vi "num2stringArr.vi"(0 "item 1":dbl, 1 "item 2":dbl, 2 "item 3":dbl, 3 "item 4":dbl, 4 "item5":dbl) -> (5 "Array":string[][](array[string]))   [LabVIEW 2015]
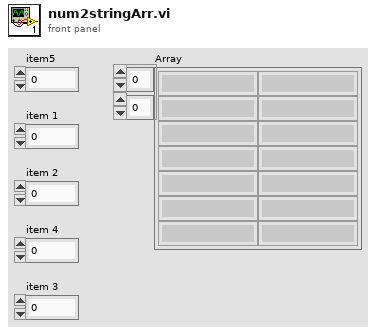
[diagram p1: front panel]
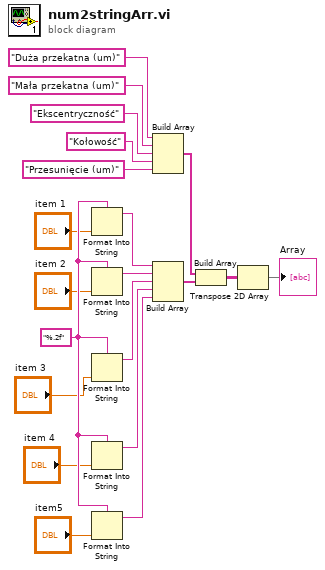
[diagram p0: block diagram]
diagram:
  w15 = "%.2f" ("format string")
  n1 = Format Into String(format string=w15, "item 1") -> (resulting string=w5:string)  [unwired: 2 in, 1 out]
  n2 = Format Into String(format string=w15, "item 2") -> (resulting string=w7:string)  [unwired: 2 in, 1 out]
  n3 = Format Into String(format string=w15, "item 3") -> (resulting string=w9:string)  [unwired: 2 in, 1 out]
  n4 = Format Into String(format string=w15, "item 4") -> (resulting string=w12:string)  [unwired: 2 in, 1 out]
  n5 = Format Into String(format string=w15, "item5") -> (resulting string=w13:string)  [unwired: 2 in, 1 out]
  n6 = Build Array("Duża przekatna (um)", "Mała przekatna (um)", "Ekscentryczność", "Kołowość", "Przesunięcie (um)") -> (w1:string[])
  n7 = Build Array(w5, w7, w9, w12, w13) -> (w2:string[])
  n8 = Build Array(w1, w2) -> (w4:string[][])
  n9 = Transpose 2D Array(2D array=w4) -> (transposed array=→"Array":string[][])
